vi "SQLite Delete Saving Goal Test.vi"(7 "Test DB Set Up Command":string, 8 "Error In (no error)":errorcluster, 11 "SQLite DB Operator In":refnum<class "SQLite DB Operator.lvclass">) -> (0 "Error Out":errorcluster, 3 "SQLite DB Operator Out":refnum<class "SQLite DB Operator.lvclass">)   [LabVIEW 2023]
uses:
  Clasess/SQLite DB Operator/SQLite DB Operator.lvclass
  Clasess/DB Records/Expenses Tracker Saving Goal/Public/Ctrls/Saving Goal.ctl
  Clasess/DB Records/Expenses Tracker Saving Goal/Expenses Tracker Saving Goal.lvclass
  H:/Desktop/LabVIEW/LabView Repo/Expenses-Tracker-DB-Operator/Interfaces/Expenses Tracker Record/Expenses Tracker Record.lvclass
  Support/Editing/Edit Record Assert Error.vi
  Support/Editing/Edit Record Assert Not Error.vi
  <vilib>/drjdpowell/SQLite Library/SQL Connection/Execute SQL (1D Cluster).vi
  <vilib>/addons/_JKI Toolkits/Caraya/classes/Test/Test.lvclass
  <vilib>/drjdpowell/SQLite Library/SQLite.lvlib
  H:/Desktop/LabVIEW/LabView Repo/Expenses-Tracker-DB-Operator/Clasess/DB Records/Expenses Tracker Saving Goal/Expenses Tracker Saving Goal.lvclass
  <vilib>/drjdpowell/SQLite Library/SQL Connection/Connection.lvclass
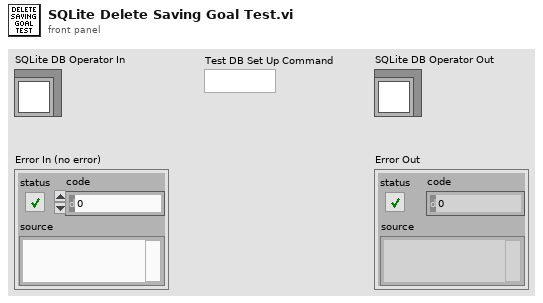
[diagram p1: front panel]
types:
  T1 = typedef "Expenses Tracker Saving Goal.lvclass/Saving Goal.ctl" = cluster{"ID":u32, "Name":string, "Current_value":dbl, "Target_value":dbl, "Date_of_entry":timestamp, "Due_date":timestamp, "Last_update":timestamp, "Description":string}
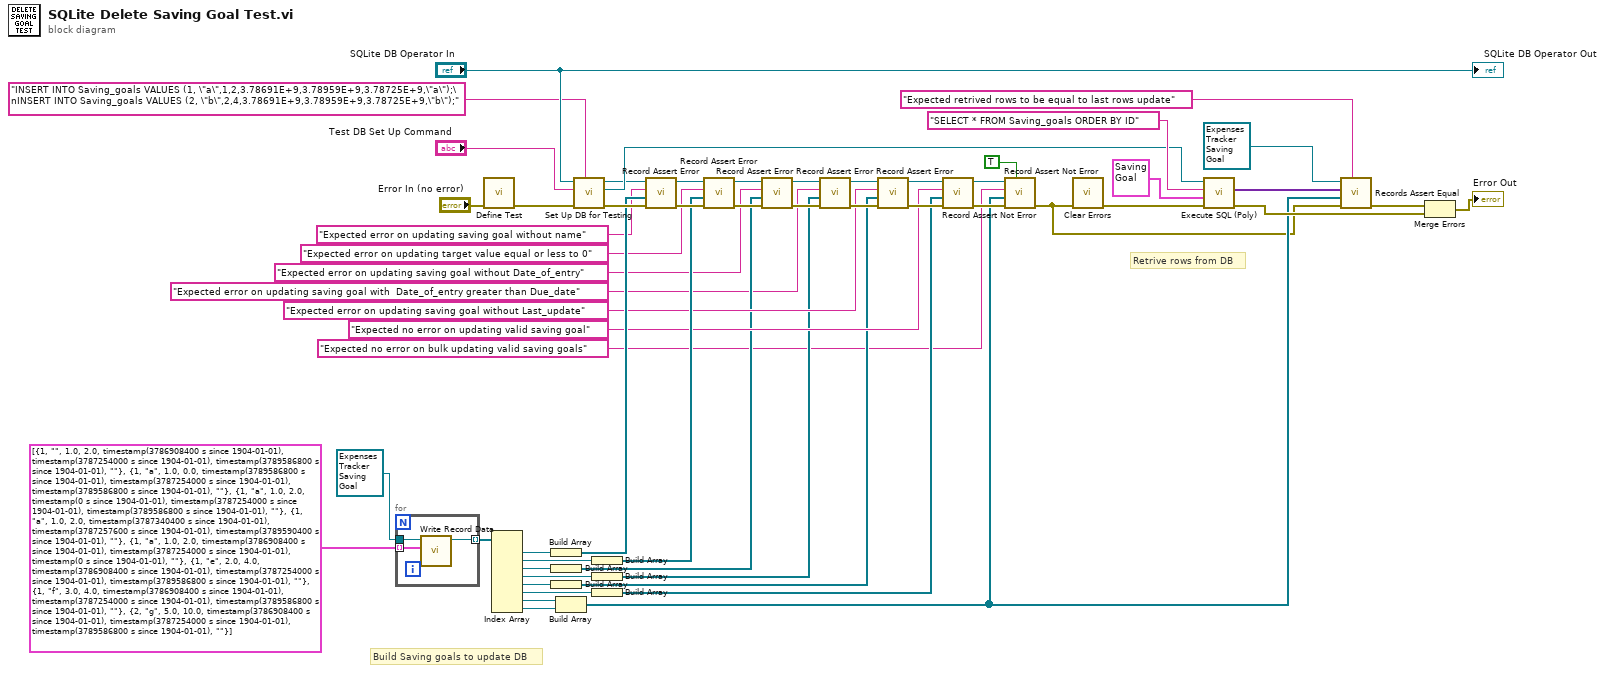
[diagram p0: block diagram]
diagram:
  # "Retrive rows from DB"
  # "Build Saving goals to update DB"
  n1 = for {
    tunnel: T1[] [{"ID"=1, "Name"="", "Current_value"=1.0, "Target_value"=2.0, "Date_of_entry"=timestamp(3786908400 s since 1904-01-01), "Due_date"=timestamp(3787254000 s since 1904-01-01), "Last_update"=timestamp(3789586800 s since 1904-01-01), "Description"=""}, {"ID"=1, "Name"="a", "Current_value"=1.0, "Target_value"=0.0, "Date_of_entry"=timestamp(3789586800 s since 1904-01-01), "Due_date"=timestamp(3787254000 s since 1904-01-01), "Last_update"=timestamp(3789586800 s since 1904-01-01), "Description"=""}, {"ID"=1, "Name"="a", "Current_value"=1.0, "Target_value"=2.0, "Date_of_entry"=timestamp(0 s since 1904-01-01), "Due_date"=timestamp(3787254000 s since 1904-01-01), "Last_update"=timestamp(3789586800 s since 1904-01-01), "Description"=""}, {"ID"=1, "Name"="a", "Current_value"=1.0, "Target_value"=2.0, "Date_of_entry"=timestamp(3787340400 s since 1904-01-01), "Due_date"=timestamp(3787257600 s since 1904-01-01), "Last_update"=timestamp(3789590400 s since 1904-01-01), "Description"=""}, {"ID"=1, "Name"="a", "Current_value"=1.0, "Target_value"=2.0, "Date_of_entry"=timestamp(3786908400 s since 1904-01-01), "Due_date"=timestamp(3787254000 s since 1904-01-01), "Last_update"=timestamp(0 s since 1904-01-01), "Description"=""}, {"ID"=1, "Name"="e", "Current_value"=2.0, "Target_value"=4.0, "Date_of_entry"=timestamp(3786908400 s since 1904-01-01), "Due_date"=timestamp(3787254000 s since 1904-01-01), "Last_update"=timestamp(3789586800 s since 1904-01-01), "Description"=""}, {"ID"=1, "Name"="f", "Current_value"=3.0, "Target_value"=4.0, "Date_of_entry"=timestamp(3786908400 s since 1904-01-01), "Due_date"=timestamp(3787254000 s since 1904-01-01), "Last_update"=timestamp(3789586800 s since 1904-01-01), "Description"=""}, {"ID"=2, "Name"="g", "Current_value"=5.0, "Target_value"=10.0, "Date_of_entry"=timestamp(3786908400 s since 1904-01-01), "Due_date"=timestamp(3787254000 s since 1904-01-01), "Last_update"=timestamp(3789586800 s since 1904-01-01), "Description"=""}] ("Array") -> [w59] mode=indexing
    tunnel: refnum<class "Expenses Tracker Saving Goal.lvclass"> refnum ("Expenses Tracker Category") -> [w57]
    tunnel: [w58] -> w54 mode=indexing
    n2 = call-dynamic "Write Record Data.vi"("Record"=w59, "Expenses Tracker Saving Goal In"=w57) -> ("Expenses Tracker Saving Goal Out"=w58:refnum<class "Expenses Tracker Saving Goal.lvclass">)  [unwired: 8 in, 1 out]
  }
  n3 = call <vilib>:"Define Test.vi"("error in (no error)"="Error In (no error)") -> ("error out"=w48:errorcluster)  [unwired: 9 in, 1 out]
  n4 = Index Array(array=w54) -> (element #1=w31:refnum<class "Expenses Tracker Saving Goal.lvclass">, element #2=w27:refnum<class "Expenses Tracker Saving Goal.lvclass">, element #3=w22:refnum<class "Expenses Tracker Saving Goal.lvclass">, element #4=w20:refnum<class "Expenses Tracker Saving Goal.lvclass">, element #5=w18:refnum<class "Expenses Tracker Saving Goal.lvclass">, element #6=w10:refnum<class "Expenses Tracker Saving Goal.lvclass">, element #7=w8:refnum<class "Expenses Tracker Saving Goal.lvclass">, element #8=w7:refnum<class "Expenses Tracker Saving Goal.lvclass">)  [unwired: 8 in]
  n5 = Build Array(w31) -> (w30:refnum<class "Expenses Tracker Saving Goal.lvclass">[])
  n6 = Build Array(w22) -> (w21:refnum<class "Expenses Tracker Saving Goal.lvclass">[])
  n7 = Build Array(w18) -> (w17:refnum<class "Expenses Tracker Saving Goal.lvclass">[])
  n8 = Build Array(w8, w7) -> (w4:refnum<class "Expenses Tracker Saving Goal.lvclass">[])
  n9 = call "Set Up DB for Testing.vi"("Additional Set Up Commands"="INSERT INTO Saving_goals VALUES (1, \"a\",1,2,3.78691E+9,3.78959E+9,3.78725E+9,\"a\");\nINSERT INTO Saving_goals VALUES (2, \"b\",2,4,3.78691E+9,3.78959E+9,3.78725E+9,\"b\");", "Error In (no error)"=w48, "Test DB Set Up Command"="Test DB Set Up Command", "SQLite DB Operator In"="SQLite DB Operator In") -> ("Error Out"=w32:errorcluster, "SQLite Connection"=w51:refnum<class "Connection.lvclass">, "SQLite DB Operator Out"=w29:refnum<class "SQLite DB Operator.lvclass">)  [unwired: 5 in]
  n10 = Build Array(w27) -> (w26:refnum<class "Expenses Tracker Saving Goal.lvclass">[])
  n11 = Build Array(w20) -> (w19:refnum<class "Expenses Tracker Saving Goal.lvclass">[])
  n12 = Build Array(w10) -> (w11:refnum<class "Expenses Tracker Saving Goal.lvclass">[])
  n13 = call-poly "Record Assert Error.vi"("Error In"=w32, "Records"=w30, "Assertion Label"="Expected error on updating saving goal without name" ("Label (VI Title)"), "SQLite DB Operator In"=w29) -> ("Error Out"=w39:errorcluster, "SQLite DB Operator Out"=w40:refnum<class "SQLite DB Operator.lvclass">)  [unwired: 6 in]
  n14 = call-poly "Record Assert Error.vi"("Error In"=w39, "Records"=w26, "Assertion Label"="Expected error on updating target value equal or less to 0" ("Label (VI Title)"), "SQLite DB Operator In"=w40) -> ("Error Out"=w37:errorcluster, "SQLite DB Operator Out"=w38:refnum<class "SQLite DB Operator.lvclass">)  [unwired: 6 in]
  n15 = call-poly "Record Assert Error.vi"("Error In"=w37, "Records"=w21, "Assertion Label"="Expected error on updating saving goal without Date_of_entry" ("Label (VI Title)"), "SQLite DB Operator In"=w38) -> ("Error Out"=w42:errorcluster, "SQLite DB Operator Out"=w41:refnum<class "SQLite DB Operator.lvclass">)  [unwired: 6 in]
  n16 = call-poly "Record Assert Error.vi"("Error In"=w42, "Records"=w19, "Assertion Label"="Expected error on updating saving goal with  Date_of_entry greater than Due_date" ("Label (VI Title)"), "SQLite DB Operator In"=w41) -> ("Error Out"=w35:errorcluster, "SQLite DB Operator Out"=w36:refnum<class "SQLite DB Operator.lvclass">)  [unwired: 6 in]
  n17 = call-poly "Record Assert Error.vi"("Error In"=w35, "Records"=w17, "Assertion Label"="Expected error on updating saving goal without Last_update" ("Label (VI Title)"), "SQLite DB Operator In"=w36) -> ("Error Out"=w33:errorcluster, "SQLite DB Operator Out"=w34:refnum<class "SQLite DB Operator.lvclass">)  [unwired: 6 in]
  n18 = call-poly "Record Assert Not Error.vi"("Error In"=w33, "Records"=w11, "Assertion Label"="Expected no error on updating valid saving goal" ("Label (VI Title)"), "SQLite DB Operator In"=w34) -> ("Error Out"=w6:errorcluster, "SQLite DB Operator Out"=w5:refnum<class "SQLite DB Operator.lvclass">)  [unwired: 6 in]
  n19 = call-poly "Record Assert Not Error.vi"("Bulk Update?"=TRUE, "Error In"=w6, "Records"=w4, "Assertion Label"="Expected no error on bulk updating valid saving goals" ("Label (VI Title)"), "SQLite DB Operator In"=w5) -> ("Error Out"=w1:errorcluster)  [unwired: 5 in, 1 out]
  n20 = call <vilib>:"Clear Errors.vi"("error in (no error)"=w1) -> ("error out"=w43:errorcluster)  [unwired: 5 in, 1 out]
  n21 = call-poly <vilib>:"Execute SQL (Poly).vi"("error in (no error)"=w43, "Cluster (or Array of Clusters)"=T1 {"ID"=0, "Name"="", "Current_value"=0.0, "Target_value"=0.0, "Date_of_entry"=timestamp(0 s since 1904-01-01), "Due_date"=timestamp(0 s since 1904-01-01), "Last_update"=timestamp(0 s since 1904-01-01), "Description"=""} ("Saving Goal"), "SQL"="SELECT * FROM Saving_goals ORDER BY ID", "SQLite Connection in"=w51) -> ("error out"=w44:errorcluster, "Result Set (Array of Clusters)"=w16:variant[])  [unwired: 5 in, 1 out]
  n22 = call "Records Assert Equal.vi"("Assertion Label"="Expected retrived rows to be equal to last rows update" ("Label (VI Title)"), "Error In"=w1, "Correct Records"=w4, "Typedef Records"=w16, "Expenses Tracker Record In"=refnum<class "Expenses Tracker Saving Goal.lvclass"> refnum ("Expenses Tracker Category")) -> ("Error Out"=w45:errorcluster)  [unwired: 6 in]
  n23 = Merge Errors(w45, w44) -> (→"Error Out":errorcluster)
  "SQLite DB Operator Out" <- "SQLite DB Operator In"
